vi "FPGA Target No IO.vi"() -> ()   [LabVIEW 2025]
uses:
  SubModules/Engine Simulation Toolkit FPGA IP/IP Source/APU/Shared Settings.ctl
  SubModules/Engine Simulation Toolkit FPGA IP/IP Source/Version Token.ctl
  SubModules/Engine Simulation Toolkit FPGA IP/IP Source/APU/Settings.ctl
  SubModules/Engine Simulation Toolkit FPGA IP/IP Source/APU/Input.ctl
  SubModules/Engine Simulation Toolkit FPGA IP/IP Source/APU/Output.ctl
  SubModules/Engine Simulation Toolkit FPGA IP/IP Source/Digital Pattern Generation/Load Input.ctl
  SubModules/Engine Simulation Toolkit FPGA IP/IP Source/Directional Speed/Load Input.ctl
  SubModules/Engine Simulation Toolkit FPGA IP/IP Source/Analog Replay/Load Input.ctl
  SubModules/Engine Simulation Toolkit FPGA IP/IP Source/Analog Replay/Settings.ctl
  SubModules/Engine Simulation Toolkit FPGA IP/IP Source/Analog Replay/Input.ctl
  SubModules/Engine Simulation Toolkit FPGA IP/IP Source/Knock Sensor/Cylinder Settings.ctl
  SubModules/Engine Simulation Toolkit FPGA IP/IP Source/Knock Sensor/Cylinder Input.ctl
  SubModules/Engine Simulation Toolkit FPGA IP/IP Source/Knock Sensor/Generate Settings.ctl
  SubModules/Engine Simulation Toolkit FPGA IP/IP Source/Knock Sensor/Generate Input.ctl
  SubModules/Engine Simulation Toolkit FPGA IP/IP Source/Digital Pattern Generation/Settings.ctl
  SubModules/Engine Simulation Toolkit FPGA IP/IP Source/Digital Pattern Generation/Input.ctl
  SubModules/Engine Simulation Toolkit FPGA IP/IP Source/Directional Speed/Settings.ctl
  SubModules/Engine Simulation Toolkit FPGA IP/IP Source/Directional Speed/Input.ctl
  SubModules/FPGA Addon Speciality IO/Source/Types/PWM.Generate.Digital.Settings.ctl
  <vilib>/Platform/TimedLoop/XDataNode/timing_clust.ctl
  <vilib>/Platform/TimedLoop/XDataNode/nitl_modes.ctl
  <vilib>/Platform/TimedLoop/XDataNode/wakeup.ctl
  <vilib>/rvi/Emulation/niFpgaSctlEmulationGetInTimedLoop.vi
  <vilib>/rvi/Emulation/niFpgaEmulationReportErrorSimple.vi
  <vilib>/rvi/Emulation/niFpgaGetClockAttributes.vi
  <vilib>/rvi/Emulation/niFpgaCriticalErrorInLSC.vi
  <vilib>/rvi/Emulation/niFpgaProcessEmulError.vi
  <vilib>/eio/utilities/niEioResolveVilibRelativePath.vi
  <vilib>/rvi/interface/RandomDataEmulation/niFpgaRandomDataHandleErrors.vi
  <vilib>/Platform/TimedLoop/XDataNode/XDataNode.xnode
  <vilib>/rvi/DataTransferAndStorage/Container/XNode/niFpgaContainer.xnode
  <vilib>/rvi/interface/RandomDataEmulation/nirviRandomDataFpgaReadWriteTemplate.vi
  <vilib>/Platform/TimedLoop/XDataNode/XDNodeRunTimeDep.lvlib
  SubModules/Engine Simulation Toolkit FPGA IP/IP Source/APU/APU.lvlib
  Templates/FPGA Wizard Templates.lvlib
  SubModules/Engine Simulation Toolkit FPGA IP/IP Source/Digital Pattern Generation/Digital Pattern Generation.lvlib
  SubModules/Engine Simulation Toolkit FPGA IP/IP Source/Directional Speed/Directional Speed.lvlib
  SubModules/Engine Simulation Toolkit FPGA IP/IP Source/Analog Replay/Analog Replay.lvlib
  SubModules/Engine Simulation Toolkit FPGA IP/IP Source/Knock Sensor/Knock Sensor.lvlib
  SubModules/FPGA Addon Speciality IO/Source/Speciality FPGA IO.lvlib
  SubModules/Engine Simulation Toolkit FPGA IP/IP Source/Engine Simulation Toolkit.lvlib
panel:
  out "Mod3.Loopback":fxp<+/-,32,8>[](array[numeric])
  out "Mod1.Monitor":bool[](array[boolean])
  in  "Accessory":bool
  in  "Key":bool
  in  "PWM Output 2.Settings":T1={"ACTIVE EDGE"=TRUE, "ACTIVE TICKS"=0, "INACTIVE TICKS"=0}
  in  "PWM Output 1.Settings":T1={"ACTIVE EDGE"=TRUE, "ACTIVE TICKS"=0, "INACTIVE TICKS"=0}
  in  "input.Crank":T2
  in  "settings.Crank":T3
  in  "input.Cam Exhaust":T4
  in  "settings.Cam Exhaust":T5
  in  "input.Cam Intake":T4
  in  "settings.Cam Intake":T5
  in  "input.Crank Temp":T4
  in  "settings.Crank Temp":T5
  out "Mod3.Monitor":fxp<+/-,32,8>[](array[numeric])
  in  "Spare AO 2":fxp<+/-,32,8> format="%#_27g"
  in  "Spare AO 1":fxp<+/-,32,8> format="%#_27g"
  in  "input.Knock 1":T6
  in  "settings.Knock 1":T7
  in  "input.Knock 1.Cylinder 6":T8={"probability compare"=65535, "high freq scaler"=0.0, "trigger position"=0}
  in  "settings.Knock 1.Cylinder 6":T9
  in  "input.Knock 1.Cylinder 5":T8={"probability compare"=65535, "high freq scaler"=0.0, "trigger position"=0}
  in  "settings.Knock 1.Cylinder 5":T9
  in  "input.Knock 1.Cylinder 4":T8={"probability compare"=65535, "high freq scaler"=0.0, "trigger position"=0}
  in  "settings.Knock 1.Cylinder 4":T9
  in  "input.Knock 1.Cylinder 3":T8={"probability compare"=65535, "high freq scaler"=0.0, "trigger position"=0}
  in  "settings.Knock 1.Cylinder 3":T9
  in  "input.Knock 1.Cylinder 2":T8={"probability compare"=65535, "high freq scaler"=0.0, "trigger position"=0}
  in  "settings.Knock 1.Cylinder 2":T9
  in  "input.Knock 1.Cylinder 1":T8={"probability compare"=65535, "high freq scaler"=0.0, "trigger position"=0}
  in  "settings.Knock 1.Cylinder 1":T9
  in  "input.Crank VR":T10
  in  "settings.Crank VR":T11
  out "Pressure 3":fxp<+/-,32,8> format="%#_27g"
  out "Pressure 2":fxp<+/-,32,8> format="%#_27g"
  out "Pressure 1":fxp<+/-,32,8> format="%#_27g"
  out "Crank VR Loopback":fxp<+/-,32,8> format="%#_27g"
  out "Mod4.Monitor":fxp<+/-,32,8>[](array[numeric])
  in  "load input.Crank VR":T12={"Data"=[0, 0, 0, 0, 0, 0, 0, 0, 0, 0, 0, 0, 0, 0, 0, 0], "LoadOffset"=0, "Done"=FALSE}
  in  "load input.Crank":T13
  in  "load input.Cam Exhaust":T14
  in  "load input.Cam Intake":T14
  in  "load input.Crank Temp":T14
  out "Actual Analog Input Loop Period (usec)":u32
  out "Actual Analog Output Loop Period (usec)":u32
  out "Actual Digital Loop Period (usec)":u32
  out "Actual DMA Loop Period (usec)":u32
  in  "Analog Input Loop Timer (uSec)":u32=10
  out "output.apu 1":T15 caption="output"
  in  "input.apu 1":T16={"desired speed"=0.0, "reset"=TRUE} caption="input"
  in  "settings.apu 1":T17 caption="settings"
  in  "est.version":T18
  in  "shared settings.apu 1":T19 {"start" format="%#.15g"}
  in  "go.apu 1":bool
  in  "Digital Loop Timer (uSec)":u32=10
  in  "Analog Output Loop Timer (uSec)":u32=10
  in  "DMA.Enable":bool
  in  "DMA.MinimumSamples":u32=100000 caption="DMA Loop Timer (uSec)"
  out "DMA.Timeout":bool
  in  "DMA.Timeout.Reset":bool
  in  "DMA Loop Timer (uSec)":u32=10
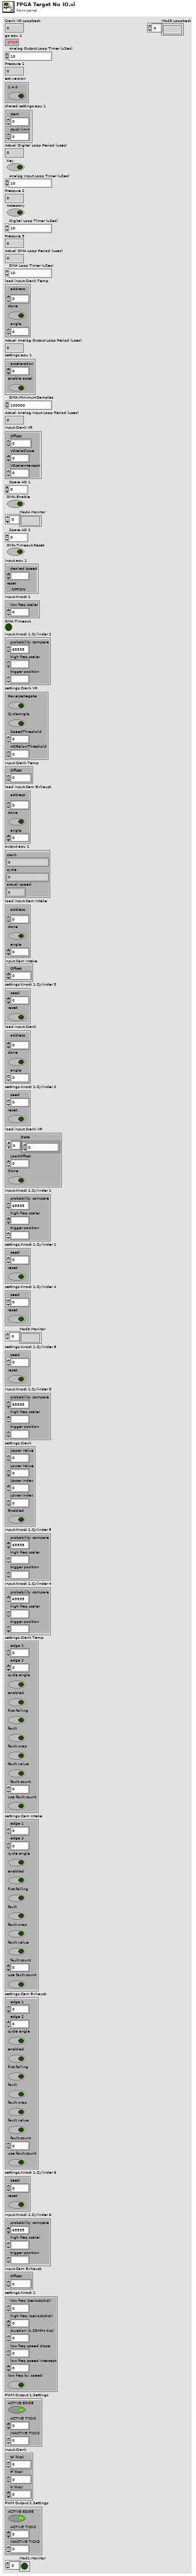
[diagram p1: front panel]
types:
  T1 = typedef "Speciality FPGA IO.lvlib/PWM.Generate.Digital.Settings.ctl" = cluster{"ACTIVE EDGE":bool, "ACTIVE TICKS":u32, "INACTIVE TICKS":u32}
  T2 = typedef "Engine Simulation Toolkit.lvlib/Directional Speed.lvlib/Input.ctl" = cluster{"td (tics)":u16, "tf (tics)":u16, "tr (tics)":u16}
  T3 = typedef "Engine Simulation Toolkit.lvlib/Directional Speed.lvlib/Settings.ctl" = cluster{"Upper Value":u16, "Lower Value":u16, "Upper Index":fxp<+,10,10>, "Lower Index":fxp<+,10,10>, "Enabled":bool}
  T4 = typedef "Engine Simulation Toolkit.lvlib/Digital Pattern Generation.lvlib/Input.ctl" = cluster{"Offset":i16}
  T5 = typedef "Engine Simulation Toolkit.lvlib/Digital Pattern Generation.lvlib/Settings.ctl" = cluster{"edge 1":u16, "edge 2":u16, "cycle angle":bool, "enabled":bool, "first falling":bool, "fault":bool, "fault wrap":bool, "fault value":bool, "fault count":fxp<+,4,4>, "use fault count":bool}
  T6 = typedef "Engine Simulation Toolkit.lvlib/Knock Sensor.lvlib/Generate Input.ctl" = cluster{"low freq scaler":fxp<+,10,0>}
  T7 = typedef "Engine Simulation Toolkit.lvlib/Knock Sensor.lvlib/Generate Settings.ctl" = cluster{"low freq (periods/tick)":fxp<+,32,0>, "high freq (periods/tick)":fxp<+,32,0>, "duration (1.25MHz tics)":fxp<+,18,18>, "low freq speed slope":fxp<+,16,-3>, "low freq speed intercept":fxp<+,10,-10>, "low freq by speed":bool}
  T8 = typedef "Engine Simulation Toolkit.lvlib/Knock Sensor.lvlib/Cylinder Input.ctl" = cluster{"probability compare":u16, "high freq scaler":fxp<+,10,0>, "trigger position":u16}
  T9 = typedef "Engine Simulation Toolkit.lvlib/Knock Sensor.lvlib/Cylinder Settings.ctl" = cluster{"seed":u16, "reset":bool}
  T10 = typedef "Engine Simulation Toolkit.lvlib/Analog Replay.lvlib/Input.ctl" = cluster{"Offset":i16, "VScaleSlope":fxp<+,18,6>, "VScaleIntercept":fxp<+/-,18,3>}
  T11 = typedef "Engine Simulation Toolkit.lvlib/Analog Replay.lvlib/Settings.ctl" = cluster{"ReverseNegate":bool, "CycleAngle":bool, "SpeedThreshold":fxp<+/-,23,2>, "AOBelowThreshold":i16}
  T12 = typedef "Engine Simulation Toolkit.lvlib/Analog Replay.lvlib/Load Input.ctl" = cluster{"Data":i16[], "LoadOffset":u16, "Done":bool}
  T13 = typedef "Engine Simulation Toolkit.lvlib/Directional Speed.lvlib/Load Input.ctl" = cluster{"address":fxp<+,10,10>, "done":bool, "angle":u16}
  T14 = typedef "Engine Simulation Toolkit.lvlib/Digital Pattern Generation.lvlib/Load Input.ctl" = cluster{"address":fxp<+,11,11>, "done":bool, "angle":u16}
  T15 = typedef "Engine Simulation Toolkit.lvlib/APU.lvlib/Output.ctl" = cluster{"crank":u16, "cycle":u16, "actual speed":fxp<+/-,23,2>}
  T16 = typedef "Engine Simulation Toolkit.lvlib/APU.lvlib/Input.ctl" = cluster{"desired speed":fxp<+/-,23,2>, "reset":bool}
  T17 = typedef "Engine Simulation Toolkit.lvlib/APU.lvlib/Settings.ctl" = cluster{"acceleration":fxp<+,18,-20>, "enable accel":bool}
  T18 = typedef "Engine Simulation Toolkit.lvlib/Version Token.ctl" = cluster{"1.4.0":bool}
  T19 = typedef "Engine Simulation Toolkit.lvlib/APU.lvlib/Shared Settings.ctl" = cluster{"start":fxp<+,17,17>, "stuck limit":fxp<+,18,18>}
  T20 = typedef "XDNodeRunTimeDep.lvlib/timing_clust.ctl" = cluster{"Expected End [f-1]":u64, "Actual End [f-1]":u64, "Finished Late? [f-1]":bool, "Expected End [i-1]":u64, "Actual End [i-1]":u64, "Finished Late? [i-1]":bool, "Expected Start [i]":u64, "Actual Start [i]":u64, "Expected Start [f]":u64, "Actual Start [f]":u64, "Source Name":string, "Structure Name":string, "Period":i64, "Deadline":i64, "Offset":i64, "Start":i64, "Priority":i32, "Timeout":i32, "Mode":T21, "Wakeup Reason":T22, "Error":errorcluster, "Source Type":string, "Secondary Source Type":string, "Global End Time":u64, "Global Start Time":u64, "Frame Duration":u64, "Iteration Duration":u64, "Assigned CPU":i32, "I/O Scan Engine Mode":u32}
  T21 = typedef "XDNodeRunTimeDep.lvlib/nitl_modes.ctl" = enum32{"No Change", "Process missed periods, maintain original phase", "Discard missed periods, maintain original phase", "Process missed periods, ignore original phase", "Discard missed periods, ignore original phase"}
  T22 = typedef "XDNodeRunTimeDep.lvlib/wakeup.ctl" = enum32{"Normal", "Aborted", "Asynchronous wakeup", "Timing source error", "Timed loop error", "Timeout"}
  T23 = typedef "Engine Simulation Toolkit.lvlib/Digital Pattern Generation.lvlib/Load Data.ctl" = cluster{"max address":fxp<+,11,11>, "memory":refnum<k21>}
  T24 = typedef "Engine Simulation Toolkit.lvlib/Directional Speed.lvlib/Load Data.ctl" = cluster{"max address":fxp<+,10,10>, "Memory":refnum<k21>}
  T25 = typedef "Engine Simulation Toolkit.lvlib/APU.lvlib/Register Bus.ctl" = cluster{"Speed":refnum<k21>, "Crank Angle":refnum<k21>, "Cycle Angle":refnum<k21>, "Crank Count":refnum<k21>, "Cycle Count":refnum<k21>, "1.25 MHz Counter":refnum<k21>, "Crank Rollover":refnum<k21>, "Cycle Rollover":refnum<k21>, "shared settings":T19}
  T26 = typedef "Engine Simulation Toolkit.lvlib/Knock Sensor.lvlib/Triggered Cylinder Data.ctl" = cluster{"trigger knock":bool, "high freq scaler":fxp<+,10,0>}
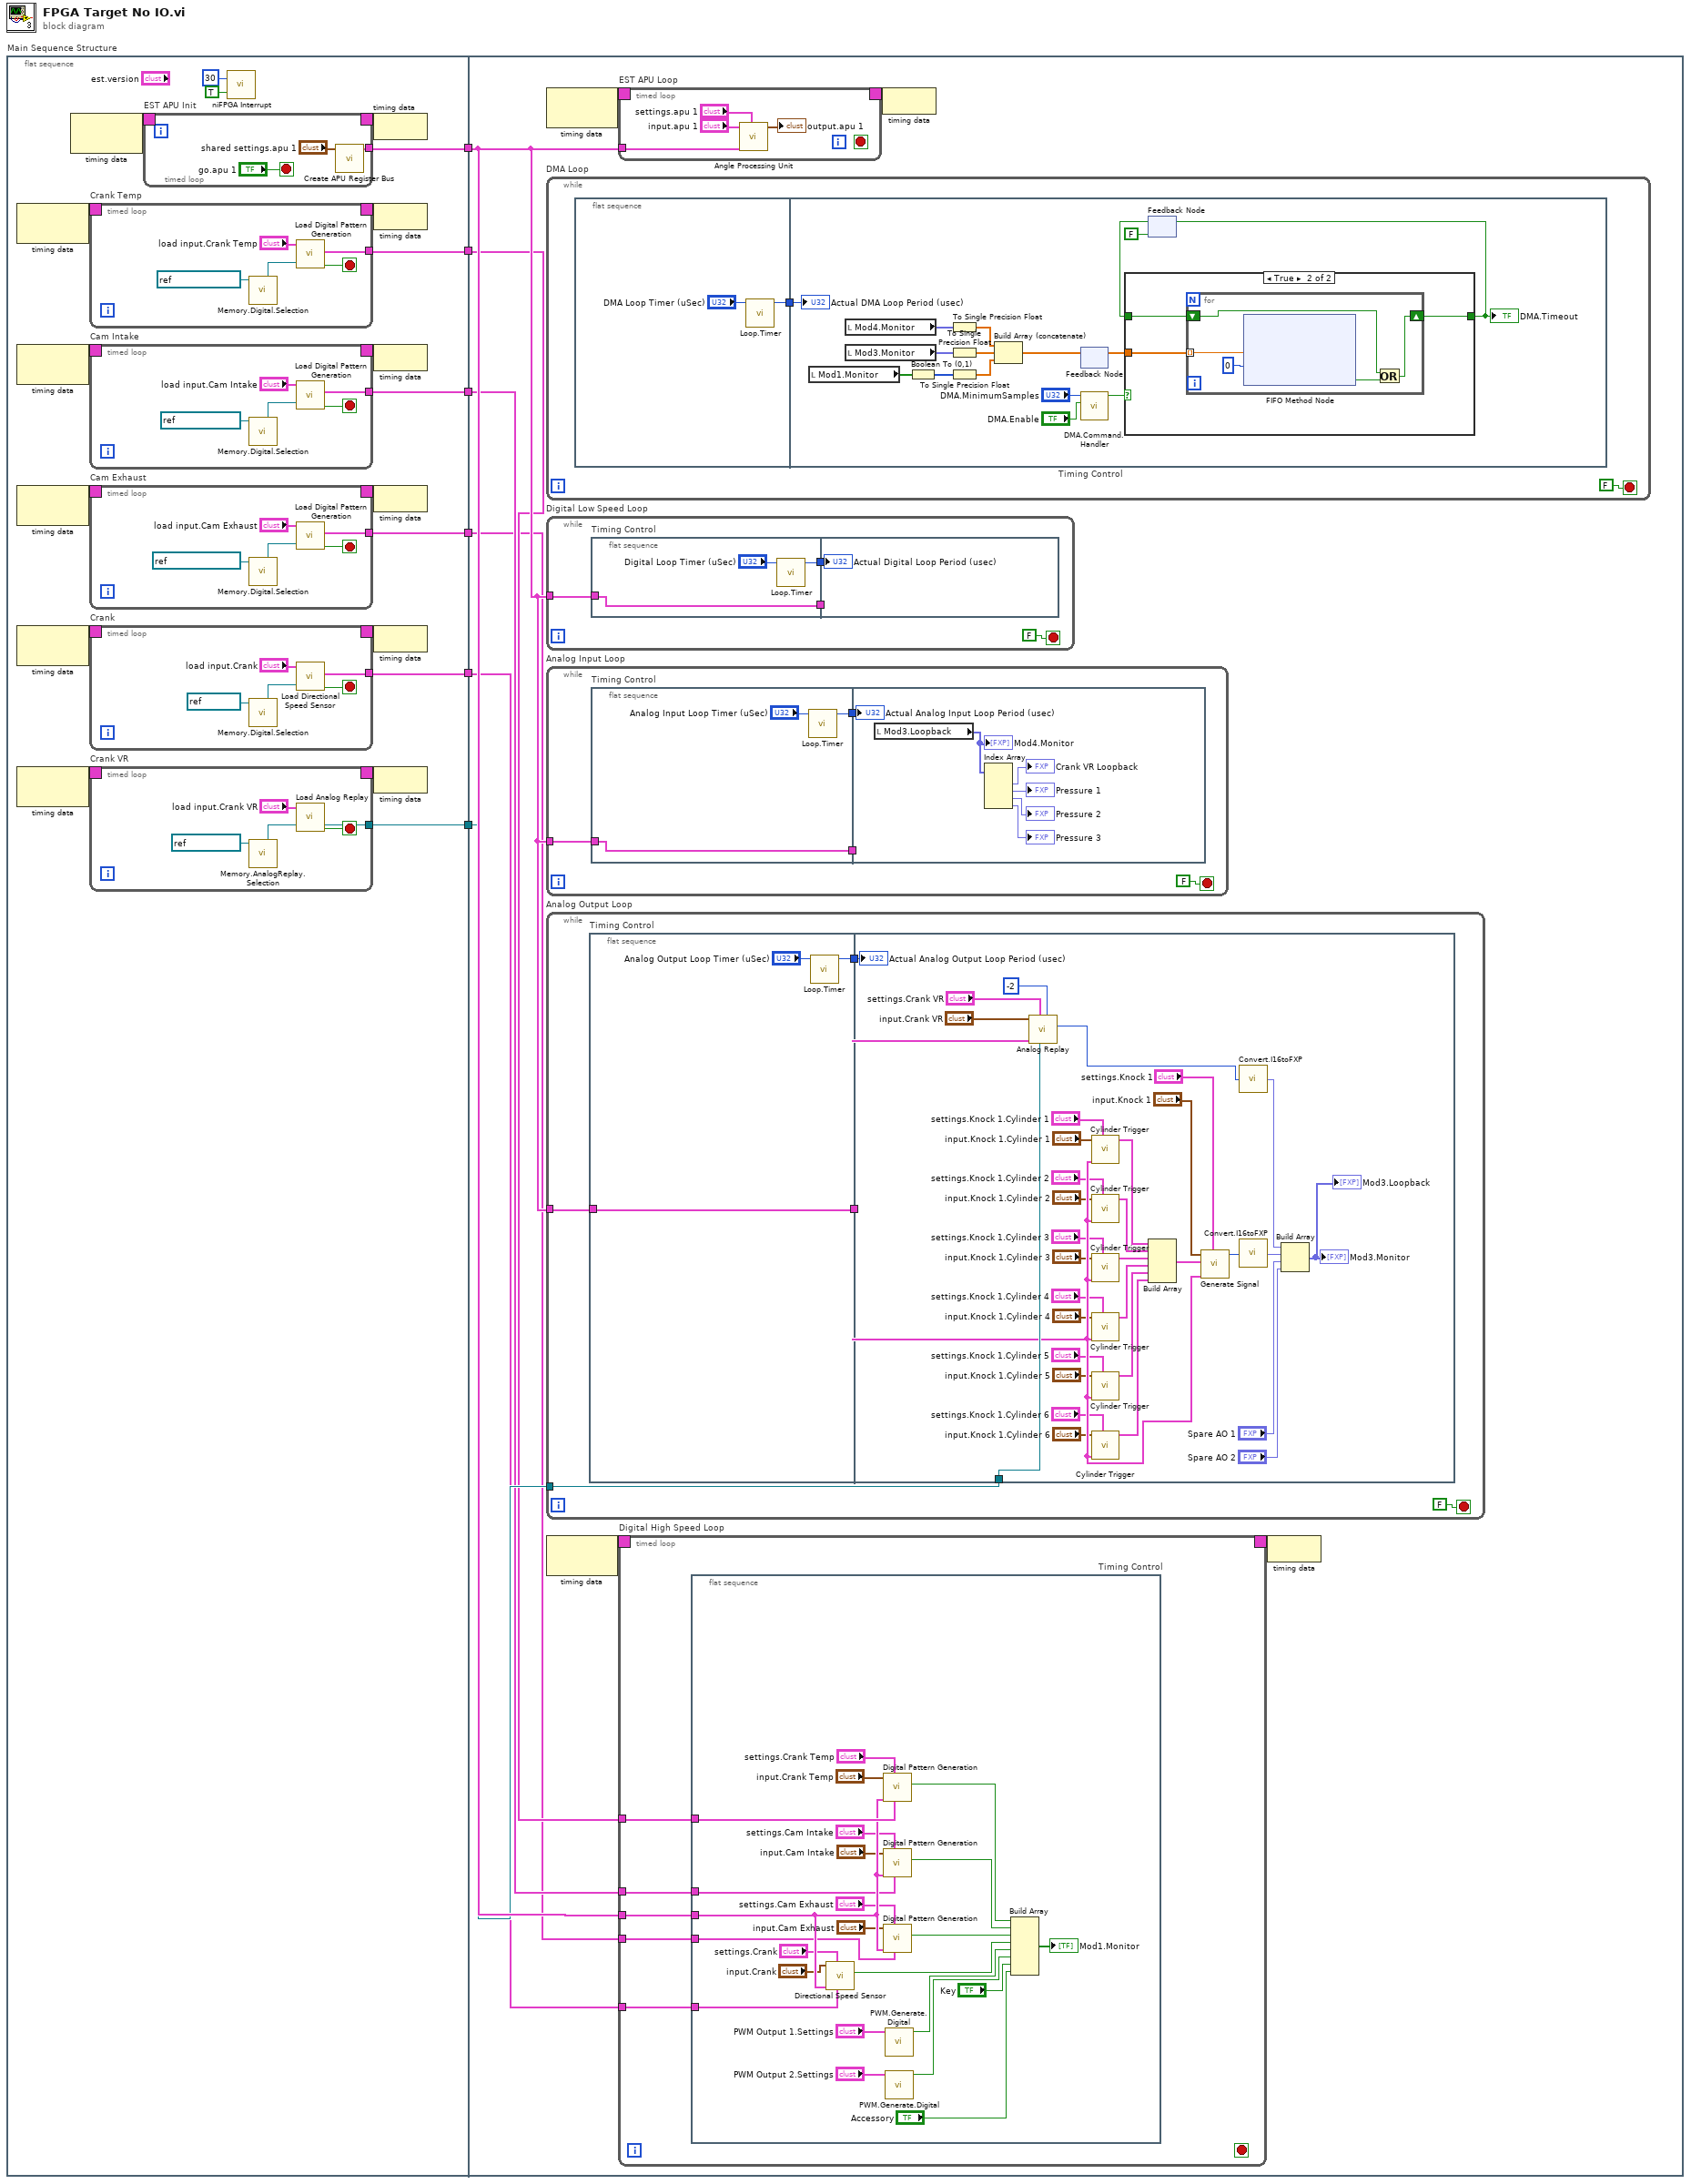
[diagram p0: block diagram]
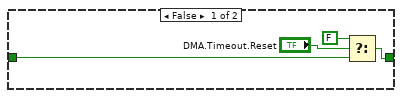
[diagram p2: hidden frame]
diagram:
  n1 = flat-sequence "Main Sequence Structure" {
    tunnel: [w22] -> w6
    tunnel: [w11] -> w5
    tunnel: [w10] -> w4
    tunnel: [w9] -> w3
    tunnel: [w8] -> w2
    tunnel: [w7] -> w1
    tunnel: w6 -> [w83]
    tunnel: w5 -> [w82]
    tunnel: w4 -> [w81]
    tunnel: w3 -> [w80]
    tunnel: w2 -> [w79]
    tunnel: w1 -> [w78]
    frame #0 {
      n2 = node-c288() -> (w21:T20)  [unwired: 1 in]
      n3 = node-c288() -> (w19:T20)  [unwired: 1 in]
      n4 = node-c288() -> (w17:T20)  [unwired: 1 in]
      n5 = node-c288() -> (w15:T20)  [unwired: 1 in]
      n6 = node-c288() -> (w13:T20)  [unwired: 1 in]
      n7 = node-c288() -> (w24:T20)  [unwired: 1 in]
      n8 = timed-loop "Crank Temp" {
        timing: w21 -> [_]
        timing-out: [_] -> w20
        tunnel: [w62] -> w10
        stop <- w65 stop-if-true
        n9 = call "Memory.Digital.Selection.vi"("memory"=refnum<k21> "Crank Temp") -> ("memory"=w63:refnum<k21>)  [unwired: 10 in]
        n10 = call "Load Digital Pattern Generation.vi"("memory"=w63, "load input.<user name>"="load input.Crank Temp") -> ("done"=w65:bool, "load data"=w62:T23)  [unwired: 8 in]
      }
      n11 = timed-loop "Cam Intake" {
        timing: w19 -> [_]
        timing-out: [_] -> w18
        tunnel: [w53] -> w9
        stop <- w56 stop-if-true
        n12 = call "Memory.Digital.Selection.vi"("memory"=refnum<k21> "Cam Intake") -> ("memory"=w54:refnum<k21>)  [unwired: 10 in]
        n13 = call "Load Digital Pattern Generation.vi"("memory"=w54, "load input.<user name>"="load input.Cam Intake") -> ("done"=w56:bool, "load data"=w53:T23)  [unwired: 8 in]
      }
      n14 = timed-loop "Cam Exhaust" {
        timing: w17 -> [_]
        timing-out: [_] -> w16
        tunnel: [w44] -> w8
        stop <- w47 stop-if-true
        n15 = call "Memory.Digital.Selection.vi"("memory"=refnum<k21> "Cam Exhaust") -> ("memory"=w45:refnum<k21>)  [unwired: 10 in]
        n16 = call "Load Digital Pattern Generation.vi"("memory"=w45, "load input.<user name>"="load input.Cam Exhaust") -> ("done"=w47:bool, "load data"=w44:T23)  [unwired: 8 in]
      }
      n17 = timed-loop "Crank" {
        timing: w15 -> [_]
        timing-out: [_] -> w14
        tunnel: [w35] -> w7
        stop <- w38 stop-if-true
        n18 = call "Memory.Digital.Selection.vi"("memory"=refnum<k21> "Crank") -> ("memory"=w36:refnum<k21>)  [unwired: 10 in]
        n19 = call "Load Directional Speed Sensor.vi"("Memory In"=w36, "load input.<user name>"="load input.Crank") -> ("done"=w38:bool, "load data"=w35:T24)  [unwired: 8 in]
      }
      n20 = timed-loop "Crank VR" {
        timing: w13 -> [_]
        timing-out: [_] -> w12
        tunnel: [w27] -> w11
        stop <- w29 stop-if-true
        n21 = call "Memory.AnalogReplay.Selection.vi"("memory"=refnum<k21> "Crank VR") -> ("memory"=w27:refnum<k21>)  [unwired: 10 in]
        n22 = call "Load Analog Replay.vi"("memory"=w27, "load input.<user name>"="load input.Crank VR") -> ("done"=w29:bool)  [unwired: 9 in]
      }
      n23 = timed-loop "EST APU Init" {
        timing: w24 -> [_]
        timing-out: [_] -> w23
        tunnel: [w71] -> w22
        stop <- "go.apu 1" stop-if-true
        n24 = call "Create APU Register Bus.vi"("shared settings.<user name>"="shared settings.apu 1") -> ("register bus"=w71:T25)  [unwired: 10 in]
      }
      n25 = call <vilib>:"niFPGA Interrupt.vi"("Wait Until Cleared (F)"=TRUE, "IRQ Number (0)"=u8 30) -> ()  [unwired: 1 in]
      n26 = node-c288(w23) -> ()
      n27 = node-c288(w20) -> ()
      n28 = node-c288(w18) -> ()
      n29 = node-c288(w16) -> ()
      n30 = node-c288(w14) -> ()
      n31 = node-c288(w12) -> ()
    }
    frame #1 {
      # "FPGA Addon Code"
      n32 = node-c288 ("Input Node")() -> (w85:T20)  [unwired: 1 in]
      n33 = while "DMA Loop" {
        stop <- FALSE stop-if-true
        n34 = flat-sequence "Timing Control" {
          tunnel: [w131] -> w129
          tunnel: w129 -> [w140]
          frame #0 {
            n35 = call "Loop.Timer.vi"("Loop Timer (uSec)"="DMA Loop Timer (uSec)") -> ("Actual Loop Period (usec)"=w131:u32)  [unwired: 10 in]
          }
          frame #1 {
            n36 = local read "Mod1.Monitor"() -> (w137:bool[])
            n37 = local read "Mod4.Monitor"() -> (w139:fxp<+/-,32,8>[])
            n38 = local read "Mod3.Monitor"() -> (w138:fxp<+/-,32,8>[])
            n39 = Boolean To (0,1)(Boolean=w137) -> (0, 1=w136:i16[])
            n40 = To Single Precision Float(number=w139) -> (single precision float=w135:sgl[])
            n41 = To Single Precision Float(number=w138) -> (single precision float=w134:sgl[])
            n42 = To Single Precision Float(number=w136) -> (single precision float=w133:sgl[])
            n43 = Build Array (concatenate) "Build Array"(w135, w134, w133) -> (w146:sgl[])
            n44 = feedback #1() -> (w145:sgl[])  [unwired: 1 in]
            n45 = feedback-in #1(w146) -> ()
            n46 = call "DMA.Command.Handler.vi"("DMA.Enable"="DMA.Enable", "DMA.MinimumSamples"="DMA.MinimumSamples") -> ("Transfer"=w142:bool)  [unwired: 9 in]
            n47 = feedback #2(FALSE ("t")) -> (w141:bool)
            n48 = case shown="True" w142 {
              tunnel: w145 -> [_ w155]
              tunnel: w141 -> [w150 w154]
              tunnel: [w149 w153] -> w144
              frame False {
                n49 = Select(t=FALSE, s="DMA.Timeout.Reset", f=w150) -> (s? t:f=w149:bool)
              }
              frame True {
                n50 = for {
                  shift-right: [w158] -> w153
                  shift-left: w154 -> [w157]
                  tunnel: w155 -> [w156] mode=indexing
                  n51 = xnode ("FIFO Method Node")("Element"=w156, "Timeout"=0) -> ("Timed Out?"=w159:bool)  [unwired: 1 in, 1 out]
                  n52 = Or(x=w157, y=w159) -> (x .or. y?=w158:bool)
                }
              }
            }
            "DMA.Timeout" <- w144
            n53 = feedback-in #2(w144) -> ()
            "Actual DMA Loop Period (usec)" <- w140
          }
        }
      }
      n54 = while "Digital Low Speed Loop" {
        tunnel: w83 -> [w218]
        stop <- FALSE stop-if-true
        n55 = flat-sequence "Timing Control" {
          tunnel: w218 -> [w222]
          tunnel: [w222] -> w217
          tunnel: [w220] -> w216
          tunnel: w217 -> [_]
          tunnel: w216 -> [w223]
          frame #0 {
            n56 = call "Loop.Timer.vi"("Loop Timer (uSec)"="Digital Loop Timer (uSec)") -> ("Actual Loop Period (usec)"=w220:u32)  [unwired: 10 in]
          }
          frame #1 {
            "Actual Digital Loop Period (usec)" <- w223
          }
        }
      }
      n57 = while "Analog Input Loop" {
        tunnel: w83 -> [w205]
        stop <- FALSE stop-if-true
        n58 = flat-sequence "Timing Control" {
          tunnel: w205 -> [w209]
          tunnel: [w209] -> w204
          tunnel: [w207] -> w203
          tunnel: w204 -> [_]
          tunnel: w203 -> [w215]
          frame #0 {
            n59 = call "Loop.Timer.vi"("Loop Timer (uSec)"="Analog Input Loop Timer (uSec)") -> ("Actual Loop Period (usec)"=w207:u32)  [unwired: 10 in]
          }
          frame #1 {
            n60 = local read "Mod3.Loopback"() -> (w210:fxp<+/-,32,8>[])
            "Mod4.Monitor" <- w210
            n61 = Index Array(array=w210) -> (element #1=→"Crank VR Loopback":fxp<+/-,32,8>, element #2=→"Pressure 1":fxp<+/-,32,8>, element #3=→"Pressure 2":fxp<+/-,32,8>, element #4=→"Pressure 3":fxp<+/-,32,8>)  [unwired: 4 in]
            "Actual Analog Input Loop Period (usec)" <- w215
          }
        }
      }
      n62 = while "Analog Output Loop" {
        tunnel: w83 -> [w164]
        tunnel: w82 -> [w161]
        stop <- FALSE stop-if-true
        n63 = flat-sequence "Timing Control" {
          tunnel: w164 -> [w168]
          tunnel: [w168] -> w163
          tunnel: [w166] -> w162
          tunnel: w163 -> [w197]
          tunnel: w162 -> [w202]
          tunnel: w161 -> [w198]
          frame #0 {
            n64 = call "Loop.Timer.vi"("Loop Timer (uSec)"="Analog Output Loop Timer (uSec)") -> ("Actual Loop Period (usec)"=w166:u32)  [unwired: 10 in]
          }
          frame #1 {
            n65 = call "Analog Replay.vi"("shift"=i8 -2, "memory"=w198, "settings.<user name>"="settings.Crank VR", "register bus"=w197, "input.<user name>"="input.Crank VR") -> ("analog value"=w196:i16)  [unwired: 6 in]
            n66 = call "Cylinder Trigger.vi"("settings.<user name>"="settings.Knock 1.Cylinder 1", "register bus"=w197, "input.<user name>"="input.Knock 1.Cylinder 1") -> ("triggered knock data"=w193:T26)  [unwired: 8 in]
            n67 = call "Cylinder Trigger.vi"("settings.<user name>"="settings.Knock 1.Cylinder 2", "register bus"=w197, "input.<user name>"="input.Knock 1.Cylinder 2") -> ("triggered knock data"=w190:T26)  [unwired: 8 in]
            n68 = call "Cylinder Trigger.vi"("settings.<user name>"="settings.Knock 1.Cylinder 3", "register bus"=w197, "input.<user name>"="input.Knock 1.Cylinder 3") -> ("triggered knock data"=w187:T26)  [unwired: 8 in]
            n69 = call "Cylinder Trigger.vi"("settings.<user name>"="settings.Knock 1.Cylinder 4", "register bus"=w197, "input.<user name>"="input.Knock 1.Cylinder 4") -> ("triggered knock data"=w184:T26)  [unwired: 8 in]
            n70 = call "Cylinder Trigger.vi"("settings.<user name>"="settings.Knock 1.Cylinder 5", "register bus"=w197, "input.<user name>"="input.Knock 1.Cylinder 5") -> ("triggered knock data"=w181:T26)  [unwired: 8 in]
            n71 = call "Cylinder Trigger.vi"("settings.<user name>"="settings.Knock 1.Cylinder 6", "register bus"=w197, "input.<user name>"="input.Knock 1.Cylinder 6") -> ("triggered knock data"=w178:T26)  [unwired: 8 in]
            n72 = Build Array(w193, w190, w187, w184, w181, w178) -> (w175:T26[])
            n73 = call "Generate Signal.vi"("settings.<user name>"="settings.Knock 1", "register bus"=w197, "triggered knock data"=w175, "input.<user name>"="input.Knock 1") -> ("knock signal"=w174:i16)  [unwired: 7 in]
            n74 = call "Convert.I16toFXP.vi"("16bit integer"=w196) -> ("x*y"=w173:fxp<+/-,20,5>)  [unwired: 4 in]
            n75 = call "Convert.I16toFXP.vi"("16bit integer"=w174) -> ("x*y"=w172:fxp<+/-,20,5>)  [unwired: 4 in]
            n76 = Build Array(w173, w172, "Spare AO 1", "Spare AO 2") -> (→"Mod3.Monitor" →"Mod3.Loopback":fxp<+/-,32,8>[])
            "Actual Analog Output Loop Period (usec)" <- w202
          }
        }
      }
      n77 = node-c288() -> (w87:T20)  [unwired: 1 in]
      n78 = timed-loop "EST APU Loop" {
        timing: w85 -> [_]
        timing-out: [_] -> w84
        tunnel: w83 -> [w88]
        stop <- _ stop-if-true
        n79 = call "Angle Processing Unit.vi"("settings.<user name>"="settings.apu 1", "register bus"=w88, "input.<user name>"="input.apu 1") -> ("output.<user name>"=→"output.apu 1":T15)  [unwired: 8 in]
      }
      n80 = timed-loop "Digital High Speed Loop" {
        timing: w87 -> [_]
        timing-out: [_] -> w86
        tunnel: w83 -> [w100]
        tunnel: w81 -> [w99]
        tunnel: w80 -> [w98]
        tunnel: w79 -> [w97]
        tunnel: w78 -> [w96]
        stop <- _ stop-if-true
        n81 = flat-sequence "Timing Control" {
          tunnel: w100 -> [w121]
          tunnel: w99 -> [w122]
          tunnel: w98 -> [w118]
          tunnel: w97 -> [w115]
          tunnel: w96 -> [w112]
          frame #0 {
            n82 = call "Directional Speed Sensor.vi"("load data"=w112, "settings.<user name>"="settings.Crank", "register bus"=w121, "input.<user name>"="input.Crank") -> ("digial output"=w106:bool)  [unwired: 7 in]
            n83 = call "Digital Pattern Generation.vi"("load data"=w122, "settings.<user name>"="settings.Crank Temp", "register bus"=w121, "input.<user name>"="input.Crank Temp") -> ("digial output"=w109:bool)  [unwired: 7 in]
            n84 = call "Digital Pattern Generation.vi"("load data"=w118, "settings.<user name>"="settings.Cam Intake", "register bus"=w121, "input.<user name>"="input.Cam Intake") -> ("digial output"=w108:bool)  [unwired: 7 in]
            n85 = call "Digital Pattern Generation.vi"("load data"=w115, "settings.<user name>"="settings.Cam Exhaust", "register bus"=w121, "input.<user name>"="input.Cam Exhaust") -> ("digial output"=w107:bool)  [unwired: 7 in]
            n86 = call "PWM.Generate.Digital.vi"("Settings"="PWM Output 1.Settings") -> ("Output"=w105:bool)  [unwired: 10 in]
            n87 = call "PWM.Generate.Digital.vi"("Settings"="PWM Output 2.Settings") -> ("Output"=w104:bool)  [unwired: 10 in]
            n88 = Build Array(w109, w108, w107, w106, w105, w104, "Key", "Accessory") -> (→"Mod1.Monitor":bool[])
          }
        }
      }
      n89 = node-c288 ("Output Node")(w84) -> ()
      n90 = node-c288 ("Output Node")(w86) -> ()
    }
  }
